vi "DMM Scan Reset_2.vi"(8 "error in (no error)":errorcluster, 11 "VISA in resource name":refnum<visa-resource-name>) -> (0 "error out":errorcluster, 3 "VISA resource name out":refnum<visa-resource-name>)   [LabVIEW 2023]
uses:
  <instrlib>/Agilent 3446X Series/Agilent 3446X Series.lvlib
panel:
  out "read buffer":string
  out "error out 4":errorcluster caption="error out"
  out "error out 3":errorcluster
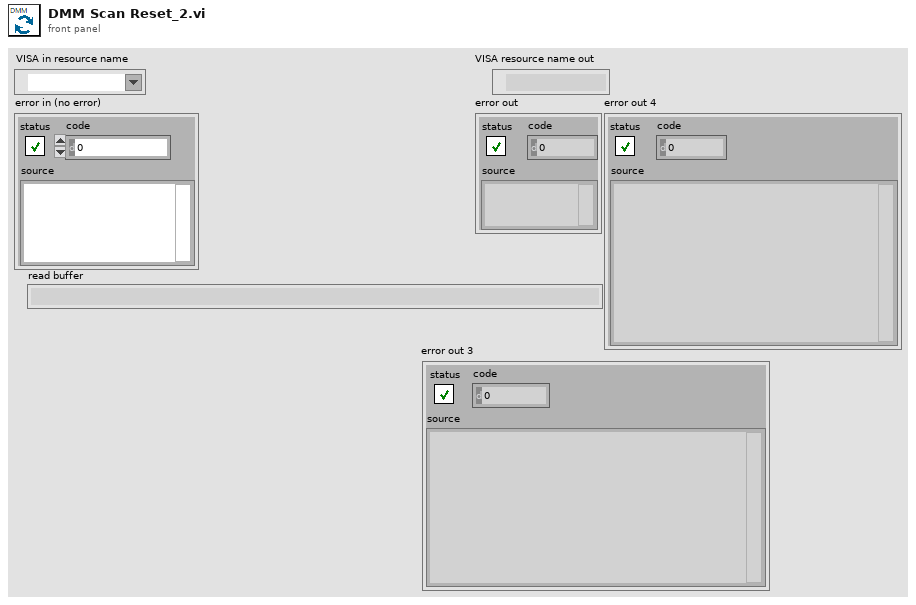
[diagram p1: front panel]
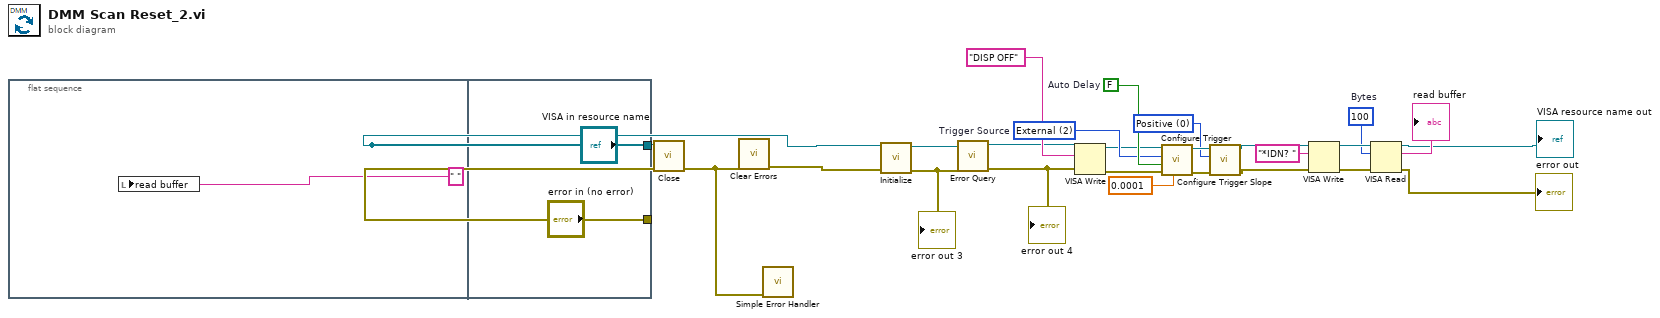
[diagram p0: block diagram]
diagram:
  w7 = u32 100  # Bytes
  w24 = 0 items=["Positive", "Negative"] ("Trigger Edge (1: Negative)")
  w22 = 2 items=["Immediate", "Software (Bus)", "External"]  # Trigger Source
  w23 = FALSE  # Auto Delay
  n1 = flat-sequence {
    tunnel: ["error in (no error)"] -> w17
    tunnel: ["VISA in resource name"] -> w11
    frame #0 {
      n2 = local write "read buffer"(" " ("read buffer")) -> ()
    }
    frame #1 {
    }
  }
  n3 = call <instrlib>:"Close.vi"("error in (no error)"=w17, "VISA resource name"=w11) -> ("error out"=w16:errorcluster)  [unwired: 9 in]
  n4 = call <vilib>:"Clear Errors.vi"("error in (no error)"=w16) -> ("error out"=w10:errorcluster)  [unwired: 5 in, 1 out]
  n5 = call <vilib>:"Simple Error Handler.vi"("error in (no error)"=w16) -> ()  [unwired: 4 in, 5 out]
  n6 = call <instrlib>:"Initialize.vi"("error in (no error)"=w10, "VISA resource name"=w11) -> ("error out"=w14:errorcluster, "VISA resource name out"=w15:refnum<visa-resource-name>)  [unwired: 3 in, 5 out]
  "error out 3" <- w14
  n7 = call <instrlib>:"Error Query.vi"("error in (no error)"=w14, "VISA resource name"=w15) -> ("error out"=w12:errorcluster, "VISA resource name out"=w13:refnum<visa-resource-name>)  [unwired: 8 out]
  "error out 4" <- w12
  n8 = VISA Write(VISA resource name=w13, write buffer="DISP OFF", error in (no error)=w12) -> (VISA resource name out=w19:refnum<visa-resource-name>, error out=w18:errorcluster)  [unwired: 1 out]
  n9 = call <instrlib>:"Configure Trigger.vi"("Manual Trigger Delay (1 s)"=0.0001, "error in (no error)"=w18, "Auto Delay (F:Disable)"=w23, "Trigger Source (0: Immediate)"=w22, "VISA resource name"=w19) -> ("error out"=w26:errorcluster, "VISA resource name out"=w25:refnum<visa-resource-name>)  [unwired: 1 in, 4 out]
  n10 = call <instrlib>:"Configure Trigger Slope.vi"("error in (no error)"=w26, "Trigger Edge (1: Negative)"=w24, "VISA resource name"=w25) -> ("error out"=w3:errorcluster, "VISA resource name out"=w4:refnum<visa-resource-name>)  [unwired: 7 in]
  n11 = VISA Write(VISA resource name=w4, write buffer="*IDN? ", error in (no error)=w3) -> (VISA resource name out=w8:refnum<visa-resource-name>, error out=w9:errorcluster)  [unwired: 1 out]
  n12 = VISA Read(VISA resource name=w8, byte count=w7, error in (no error)=w9) -> (VISA resource name out=→"VISA resource name out":refnum<visa-resource-name>, read buffer=→"read buffer":string, error out=→"error out":errorcluster)  [unwired: 1 out]
